vi "OPCUA Connect.vi"(8 "error in (no error)":errorcluster, 9 "sDataDir":string, 10 "ipAddr":string) -> (0 "error out":errorcluster, 1 "ExitCode":i32(ring) items=["Ok"=0, "ErrorCreateApplication"=17, "ErrorDiscoverEndpoints"=18, "ErrorCreateSession"=19, "ErrorBrowseNamespace"=20, "ErrorCreateSubscription"=21, "ErrorMonitoredItem"=22, "ErrorAddSubscription"=23, "ErrorRunning"=24, "ErrorNoKeepAlive"=48, "ErrorNoSecurityFile"=49, "ErrorInvalidCommandLine"=256], 2 "Handle":refnum<k24>)   [LabVIEW 2019]
uses:
  F:/src/HUTCDLSVN/Machine/CDL0100/TagEngine/LVOPCUA.NET/LVOPC.NETInterface/bin/Release/LVOPC.NETInterface.dll
  LVOPCUA.NET/LVOPC.NETInterface/bin/Release/LVOPC.NETInterface.dll
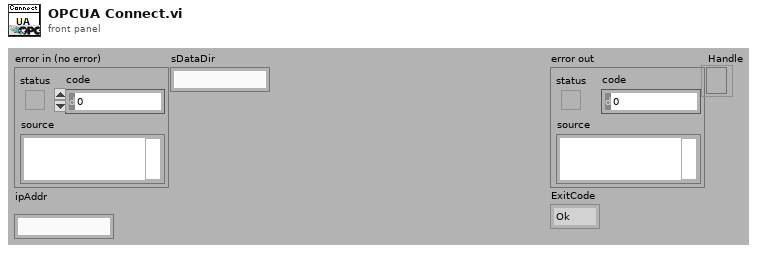
[diagram p1: front panel]
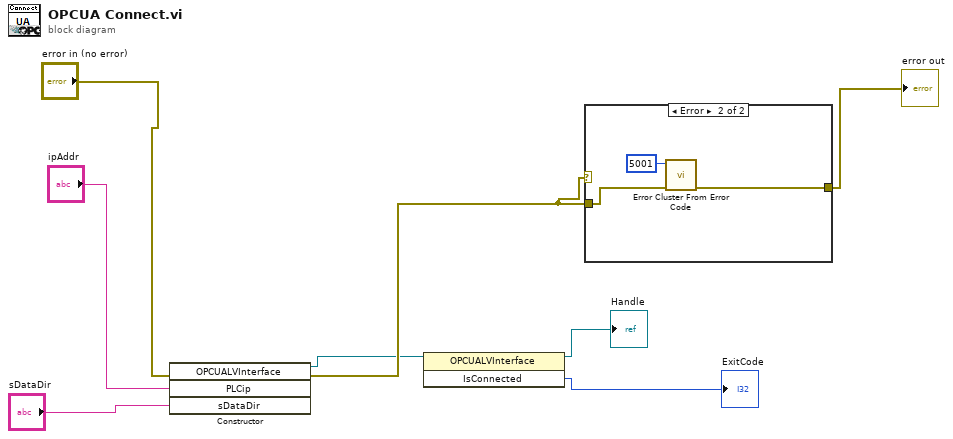
[diagram p0: block diagram]
diagram:
  n1 = constructor class="OPCUALVInterface"(error in="error in (no error)", "PLCip"="ipAddr", "sDataDir"="sDataDir") -> (reference out=w3:refnum<k24>, error out=w5:errorcluster)  [unwired: 2 in, 3 out]
  n2 = invoke class="OPCUALVInterface" method="IsConnected"(reference=w3) -> (reference out=→"Handle":refnum<k24>, "IsConnected"=→"ExitCode":i32)  [unwired: 2 in, 1 out]
  n3 = case shown="Error" w5 {
    tunnel: [w9 w11] -> w8
    tunnel: w5 -> [w9 w10]
    frame No Error {
    }
    frame Error {
      n4 = call <vilib>:"Error Cluster From Error Code.vi"("error in (no error)"=w10, "error code (0)"=5001) -> ("error out"=w11:errorcluster)  [unwired: 7 in]
    }
  }
  "error out" <- w8
